vi "Primary Driver.vi"(6 "Primary Driver":T1, 7 "Secondary Driver":T1, 8 "Teleop Seconds":dbl) -> (1 "Driver":dbl=0.1 format="%#_13g")   [LabVIEW 2014]
uses:
  Team Code/Robot Global Data.vi
panel:
  in  "Left Motor Scale":dbl=1.0 format="%#_13g"
  in  "Tolerance":dbl=2.0 format="%#_13g"
  in  "Y Tolerance for Quick Turn":dbl=0.5 format="%#_13g"
  in  "X Tolerance for Quick Turn":dbl=0.5 format="%#_13g"
  in  "Time Delay":dbl=0.25 format="%#_13g"
  in  "Min. Power":dbl=0.1 format="%#_13g"
  in  "Timer Variable":dbl
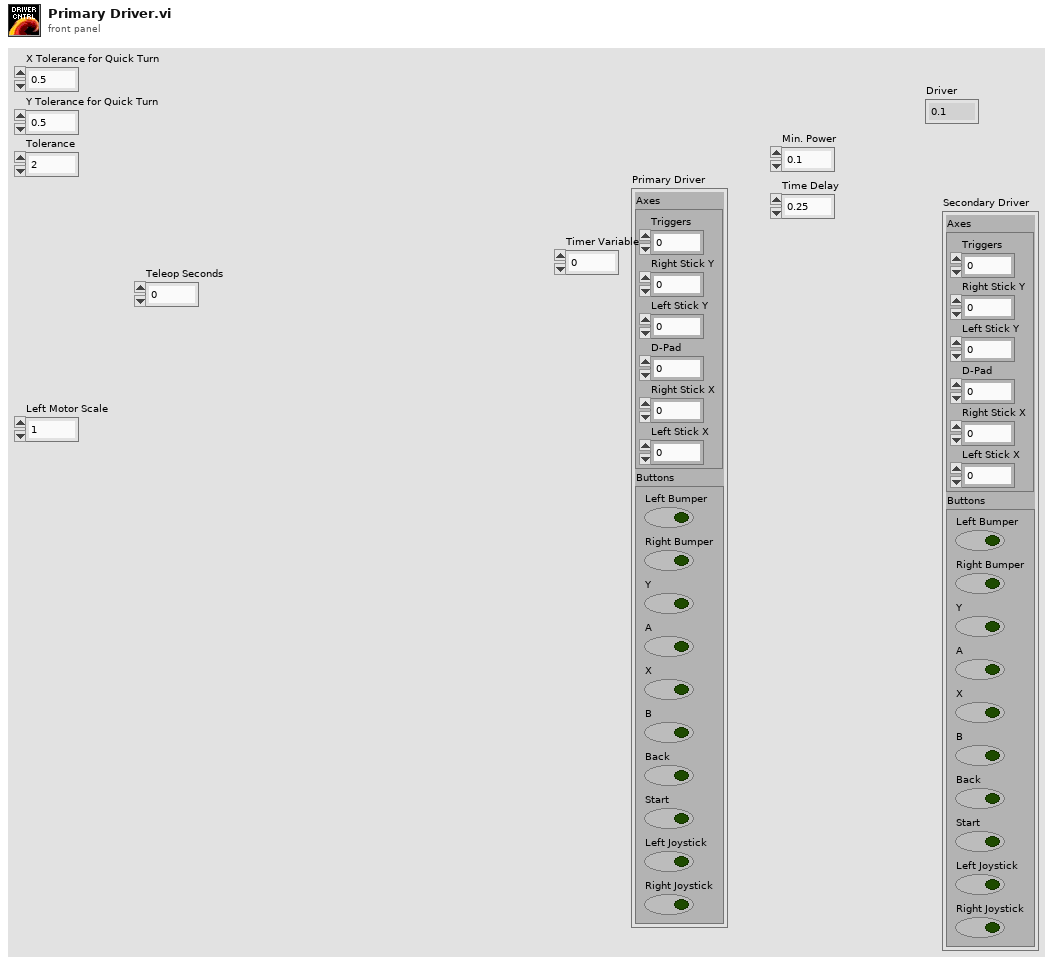
[diagram p1: front panel]
types:
  T1 = cluster{"Axes":cluster{"Triggers":dbl, "Right Stick Y":dbl, "Left Stick Y":dbl, "D-Pad":dbl, "Right Stick X":dbl, "Left Stick X":dbl}, "Buttons":cluster{"Left Bumper":bool, "Right Bumper":bool, "Y":bool, "A":bool, "X":bool, "B":bool, "Back":bool, "Start":bool, "Left Joystick":bool, "Right Joystick":bool}}
  T2 = cluster{"FIRE!!!":bool, "Loader":bool, "Lock":bool, "Load":bool, "Pass":bool, "Grab":bool, "PANIC":bool, "Don't Cock":bool, "Roller Speed":dbl}
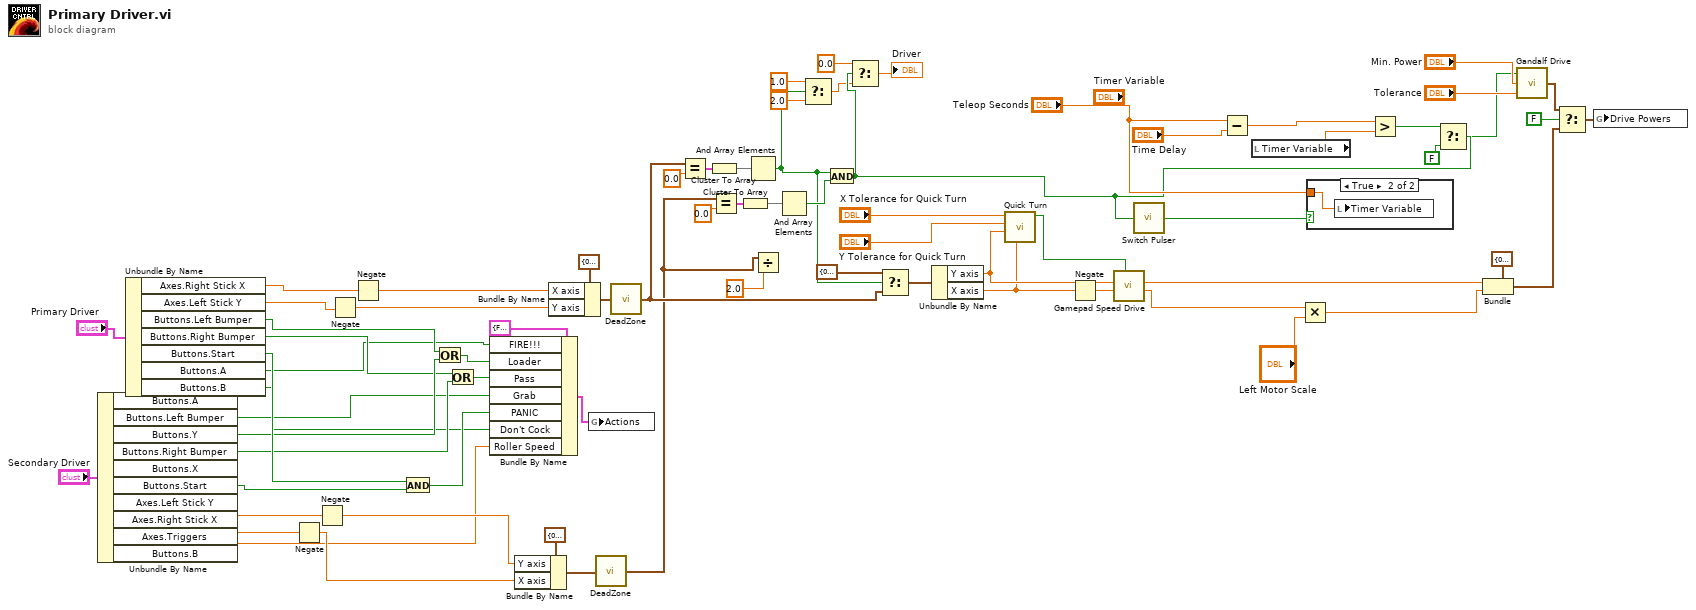
[diagram p0: block diagram]
diagram:
  n1 = Unbundle By Name("Secondary Driver") -> ("Buttons.Left Bumper"=w12:bool, "Buttons.Y"=w17:bool, "Buttons.Right Bumper"=w15:bool, "Buttons.Start"=w46:bool, "Axes.Left Stick Y"=w43:dbl, "Axes.Right Stick X"=w42:dbl, "Axes.Triggers"=w7:dbl)  [unwired: 3 out]
  n2 = Unbundle By Name("Primary Driver") -> ("Axes.Right Stick X"=w51:dbl, "Axes.Left Stick Y"=w53:dbl, "Buttons.Left Bumper"=w18:bool, "Buttons.Right Bumper"=w16:bool, "Buttons.Start"=w49:bool, "Buttons.A"=w1:bool, "Buttons.B"=w3:bool)
  n3 = Negate(x=w42) -> (-x=w40:dbl)
  n4 = Negate(x=w43) -> (-x=w41:dbl)
  n5 = Negate(x=w53) -> (-x=w52:dbl)
  n6 = Negate(x=w51) -> (-x=w54:dbl)
  n7 = And(x=w49, y=w46) -> (x .and. y?=w48:bool)
  n8 = Or(x=w18, y=w17) -> (x .or. y?=w14:bool)
  n9 = Or(x=w16, y=w15) -> (x .or. y?=w13:bool)
  n10 = Bundle By Name(cluster=T2 {"FIRE!!!"=FALSE, "Loader"=FALSE, "Lock"=FALSE, "Load"=FALSE, "Pass"=FALSE, "Grab"=FALSE, "PANIC"=FALSE, "Don't Cock"=FALSE, "Roller Speed"=0.0} ("Actions"), "FIRE!!!"=w1, "Loader"=w14, "Pass"=w13, "Grab"=w12, "PANIC"=w48, "Don't Cock"=w3, "Roller Speed"=w7) -> (w8:T2)
  n11 = Bundle By Name(cluster=cluster{"X axis":dbl, "Y axis":dbl} {"X axis"=0.0, "Y axis"=0.0} ("Drive Axes"), "Y axis"=w41, "X axis"=w40) -> (w44:cluster{"X axis":dbl, "Y axis":dbl})
  n12 = Bundle By Name(cluster=cluster{"X axis":dbl, "Y axis":dbl} {"X axis"=0.0, "Y axis"=0.0} ("Drive Axes"), "X axis"=w54, "Y axis"=w52) -> (w71:cluster{"X axis":dbl, "Y axis":dbl})
  n13 = global write "Robot Global Data.vi" "Actions"(w8) -> ()
  n14 = call "DeadZone.vi"("Drive Axes"=w44) -> ("Drive Axes"=w11:cluster{"X axis":dbl, "Y axis":dbl})
  n15 = call "DeadZone.vi"("Drive Axes"=w71) -> ("Drive Axes"=w34:cluster{"X axis":dbl, "Y axis":dbl})
  n16 = Equal?(x=w34, y=0.0 ("X axis")) -> (x = y?=w64:cluster{"X axis":bool, "Y axis":bool})
  n17 = Cluster To Array(cluster=w64) -> (array=w63:bool[])
  n18 = Equal?(x=w11, y=0.0 ("X axis")) -> (x = y?=w38:cluster{"X axis":bool, "Y axis":bool})
  n19 = Cluster To Array(cluster=w38) -> (array=w39:bool[])
  n20 = And Array Elements(Boolean array=w63) -> (logical AND=w29:bool)
  n21 = Divide(x=w11, y=2.0 ("X axis")) -> ()  [unwired: 1 out]
  n22 = And Array Elements(Boolean array=w39) -> (logical AND=w36:bool)
  n23 = Select(t=1.0, s=w29, f=2.0) -> (s? t:f=w30:dbl)
  n24 = And(x=w29, y=w36) -> (x .and. y?=w32:bool)
  n25 = Select(t=0.0, s=w32, f=w30) -> (s? t:f=→"Driver":dbl)
  n26 = Select(t=cluster{"X axis":dbl, "Y axis":dbl} {"X axis"=0.0, "Y axis"=0.0}, s=w29, f=w34) -> (s? t:f=w33:cluster{"X axis":dbl, "Y axis":dbl})
  n27 = Unbundle By Name(w33) -> ("Y axis"=w50:dbl, "X axis"=w21:dbl)
  n28 = call "Quick Turn"("X axis"=w21, "Y axis"=w50, "Y Tolerance for Quick Turn"="Y Tolerance for Quick Turn", "X Tolerance for Quick Turn"="X Tolerance for Quick Turn") -> ("Quick Turn?"=w58:bool)  [unwired: 7 in]
  n29 = Negate(x=w21) -> (-x=w20:dbl)
  n30 = call "Gamepad Speed Drive.vi"("Quick Turn"=w58, "Turn"=w20, "Speed"=w50) -> ("Right Output"=w6:dbl, "Left Output"=w24:dbl)  [unwired: 7 in]
  n31 = call "Switch Pulser.vi"("Boolean"=w32) -> ("Boolean 2"=w62:bool)
  n32 = Subtract(x="Teleop Seconds", y="Time Delay") -> (x-y=w60:dbl)
  n33 = local read "Timer Variable"() -> (w69:dbl)
  n34 = Multiply(x=w6, y="Left Motor Scale") -> (x*y=w4:dbl)
  n35 = case shown="True" w62 {
    tunnel: "Teleop Seconds" -> [_ w74]
    frame False {
    }
    frame True {
      n36 = local write "Timer Variable"(w74) -> ()
    }
  }
  n37 = Greater?(x=w60, y=w69) -> (0:w68:bool)
  n38 = Select(t=w68, s=w32, f=FALSE) -> (s? t:f=w23:bool)
  n39 = Bundle(cluster=cluster{"RMotor":dbl, "LMotor":dbl} {"RMotor"=0.0, "LMotor"=0.0}, "RMotor"=w24, "LMotor"=w4) -> (w19:cluster{"RMotor":dbl, "LMotor":dbl})
  n40 = call "Gandalf Drive.vi"("Tolerance"="Tolerance", "Min. Power"="Min. Power", "Reset"=w23) -> ("Motor Powers"=w66:cluster{"RMotor":dbl, "LMotor":dbl})
  n41 = Select(t=w66, s=FALSE, f=w19) -> (s? t:f=w55:cluster{"RMotor":dbl, "LMotor":dbl})
  n42 = global write "Robot Global Data.vi" "Drive Powers"(w55) -> ()
